vi "getPositionersList.vi"(8 "error in":errorcluster, 11 "connection ID":refnum<k5>) -> (0 "error out":errorcluster, 2 "Positioners List":string[](array[string]), 3 "connection ID":refnum<k5>)   [LabVIEW 2016]
panel:
  in  "Get Command":string="com.attocube.amc.description.getPositionersList"
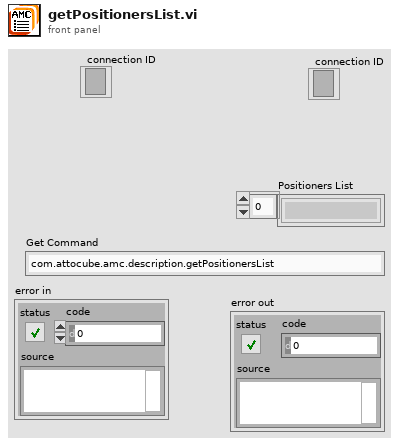
[diagram p1: front panel]
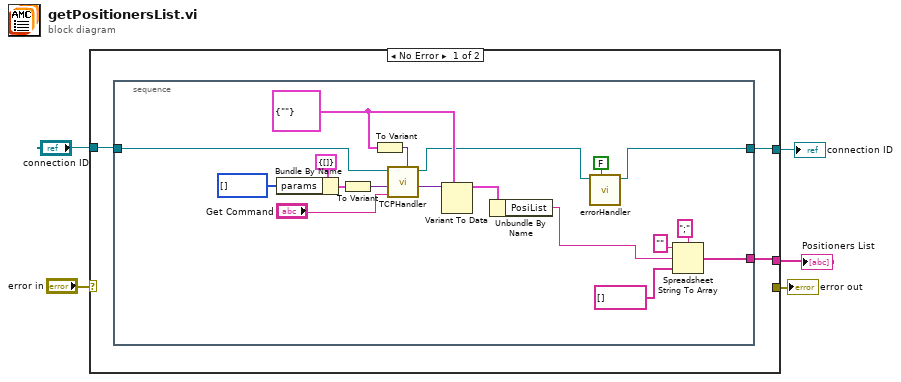
[diagram p0: block diagram]
diagram:
  n1 = case shown="No Error" "error in" {
    selector: "error in" -> [_ w28]
    tunnel: [_ w28] -> w5
    tunnel: "connection ID" -> [w8 w27]
    tunnel: [w6 w27] -> w3
    tunnel: [w7 _] -> w2
    frame No Error {
      n2 = stacked-sequence {
        tunnel: [w15] -> w6
        tunnel: w8 -> [w20]
        tunnel: [w11] -> w7
        frame #0 {
          w18 = cluster{"PosiList":string} {"PosiList"=""} ("input cluster")
          n3 = Bundle By Name(cluster=cluster{"params":i16[]} {"params"=[]} ("input cluster"), "params"=i16[] []) -> (w24:cluster{"params":i16[]})
          n4 = To Variant(anything=w24) -> (Variant=w25:variant)
          n5 = To Variant(anything=w18) -> (Variant=w19:variant)
          n6 = call "TCPHandler.vi"("result Types"=w19, "method"="Get Command", "params"=w25, "connection ID"=w20) -> ("result"=w22:variant, "connection ID"=w16:refnum<k5>)  [unwired: 5 in, 1 out]
          n7 = Variant To Data(type=w18, Variant=w22) -> (data=w26:cluster{"PosiList":string})  [unwired: 1 in, 1 out]
          n8 = Unbundle By Name(w26) -> ("PosiList"=w9:string)
          n9 = call "errorHandler.vi"("show popup"=FALSE, "connection ID"=w16) -> ("connection ID"=w15:refnum<k5>)  [unwired: 8 in, 1 out]
          n10 = Spreadsheet String To Array(delimiter (Tab)=";", format string="", spreadsheet string=w9, array type (2D Dbl)=string[] []) -> (array=w11:string[])
        }
      }
    }
    frame Error {
    }
  }
  "error out" <- w5
  "connection ID" <- w3
  "Positioners List" <- w2
